vi "Begin_ConveyorV2.vi"() -> (0 "error out":errorcluster)   [LabVIEW 2012]
uses:
  <vilib>/Rock Robotics/SystemInterfaces/Typedef/FPGA_TypedefDigitalModule.ctl
  <vilib>/Rock Robotics/SystemInterfaces/DIO/FPGA_DIOChannel.ctl
  <vilib>/Rock Robotics/WPI/CAN/Jaguar/SubVIs/WPI_CANJaguar_BrakeCoastMode.ctl
  <vilib>/Rock Robotics/WPI/MotorControl/WPI_MotorControlOpenCANJaguar.vi
  <vilib>/Rock Robotics/SystemInterfaces/AI/FPGA_AIChannel.ctl
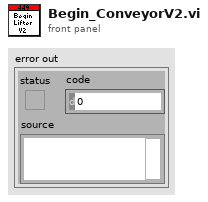
[diagram p1: front panel]
types:
  T1 = typedef "WPI_CANJaguar_BrakeCoastMode.ctl" = enum8{"Jumper", "Brake", "Coast"}
  T2 = typedef "WPI_MotorControlDeviceRef.ctl" = cluster{"DeviceStatus":errorcluster, "Type":enum16{"PWM", "CAN"}, "PWM":cluster{"Digital Module":T3, "PWM Channel":T4, "DeadBand":T5}, "CAN":cluster{"Device Number":u8, "Control Mode":T6, "Semaphore":T7, "Max Vout":dbl}, "Invert":bool, "TransformRef":T8, "InvTransformRef":T8}
  T3 = typedef "FPGA_TypedefDigitalModule.ctl" = enum16{"Digital Module 1", "Digital Module 2"}
  T4 = typedef "FPGA_DIOPWMChannel.ctl" = enum8{"PWM 1", "PWM 2", "PWM 3", "PWM 4", "PWM 5", "PWM 6", "PWM 7", "PWM 8", "PWM 9", "PWM 10", "Invalid"}
  T5 = typedef "WPI_PWMDeadband.ctl" = cluster{"Name":string, "maxPositivePwm":i32, "minPositivePwm":i32, "centerPwm":i32, "maxNegativePwm":i32, "minNegativePwm":i32, "angularRange":u16}
  T6 = typedef "WPI_CANJaguar_ControlMode.ctl" = enum8{"Percent VBus", "Current", "Speed", "Position", "Voltage"}
  T7 = typedef "Semaphore RefNum" = refnum<k1>
  T8 = typedef "WPI_PWMTransform_ConPane.ctl" = refnum<vi>
  T9 = typedef "FPGA_AIChannel.ctl" = enum8{"AI 1", "AI 2", "AI 3", "AI 4", "AI 5", "AI 6", "AI 7", "AI 8", "Invalid"}
  T10 = typedef "FPGA_DIOChannel.ctl" = enum8{"DIO 1", "DIO 2", "DIO 3", "DIO 4", "DIO 5", "DIO 6", "DIO 7", "DIO 8", "DIO 9", "DIO 10", "DIO 11", "DIO 12", "DIO 13", "DIO 14", "Invalid"}
  T11 = typedef "WPI_DigitalInputDevRef.ctl" = cluster{"DevStatus":errorcluster, "DIO Channel":T10, "Digital Module":T3}
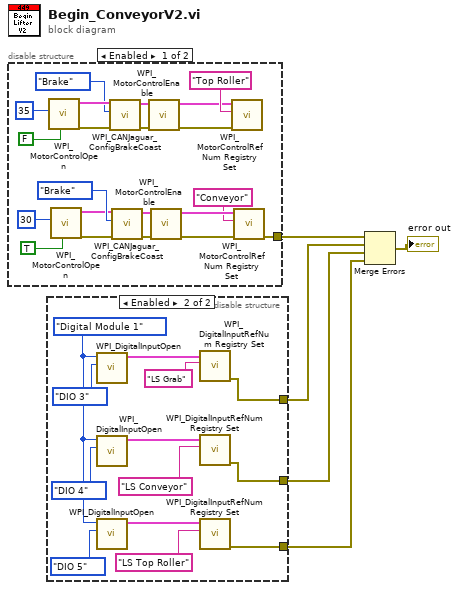
[diagram p0: block diagram]
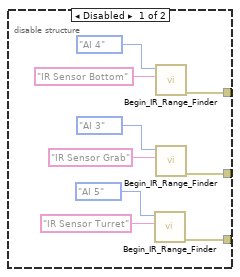
[diagram p2: hidden frame]
diagram:
  n1 = disable-structure shown="Enabled" {
    disable-tunnel: [w16 _] -> w4
    frame Enabled {
      n2 = call-poly <vilib>:"WPI_MotorControlOpen.vi"("Invert"=FALSE, "Device Number"=u8 35) -> ("error out"=w7:errorcluster, "MotorControlDeviceRef"=w8:T2)  [unwired: 8 in]
      n3 = call-poly <vilib>:"WPI_MotorControlOpen.vi"("Invert"=TRUE, "Device Number"=u8 30) -> ("error out"=w25:errorcluster, "MotorControlDeviceRef"=w24:T2)  [unwired: 8 in]
      n4 = call <vilib>:"WPI_CANJaguar_ConfigBrakeCoast.vi"("error in (no error)"=w7, "Brake / Coast Mode"=WPI_CANJaguar_BrakeCoastMode."Brake", "CAN Jaguar Ref"=w8) -> ("error out"=w10:errorcluster, "CAN Jaguar Ref Out"=w9:T2)  [unwired: 7 in]
      n5 = call <vilib>:"WPI_CANJaguar_ConfigBrakeCoast.vi"("error in (no error)"=w25, "Brake / Coast Mode"=WPI_CANJaguar_BrakeCoastMode."Brake", "CAN Jaguar Ref"=w24) -> ("error out"=w22:errorcluster, "CAN Jaguar Ref Out"=w23:T2)  [unwired: 7 in]
      n6 = call <vilib>:"WPI_MotorControlEnable.vi"("error in (no error)"=w10, "CAN Jaguar Ref"=w9) -> ("error out"=w15:errorcluster, "CAN Jaguar Ref Out"=w13:T2)  [unwired: 8 in]
      n7 = call <vilib>:"WPI_MotorControlEnable.vi"("error in (no error)"=w22, "CAN Jaguar Ref"=w23) -> ("error out"=w17:errorcluster, "CAN Jaguar Ref Out"=w19:T2)  [unwired: 8 in]
      n8 = call <vilib>:"WPI_MotorControlRefNum Registry Set.vi"("error in (no error)"=w15, "refnum name"="Top Roller", "MotorControlDevRef"=w13) -> ()  [unwired: 7 in, 2 out]
      n9 = call <vilib>:"WPI_MotorControlRefNum Registry Set.vi"("error in (no error)"=w17, "refnum name"="Conveyor", "MotorControlDevRef"=w19) -> ("error out"=w16:errorcluster)  [unwired: 7 in, 1 out]
    }
    frame Disabled {
    }
  }
  n10 = disable-structure shown="Enabled" {
    disable-tunnel: [w35 w44] -> w3
    disable-tunnel: [w34 w43] -> w2
    disable-tunnel: [w31 w42] -> w1
    frame Disabled {
      n11 = call "Begin_IR_Range_Finder.vi"("Reference Name"="IR Sensor Turret", "Analog Channel"=FPGA_AIChannel."AI 5") -> ("error out"=w31:errorcluster)  [unwired: 9 in]
      n12 = call "Begin_IR_Range_Finder.vi"("Reference Name"="IR Sensor Bottom", "Analog Channel"=FPGA_AIChannel."AI 4") -> ("error out"=w35:errorcluster)  [unwired: 9 in]
      n13 = call "Begin_IR_Range_Finder.vi"("Reference Name"="IR Sensor Grab", "Analog Channel"=FPGA_AIChannel."AI 3") -> ("error out"=w34:errorcluster)  [unwired: 9 in]
    }
    frame Enabled {
      w48 = FPGA_TypedefDigitalModule."Digital Module 1" ("Digital Module (Module 1)")
      n14 = call <vilib>:"WPI_DigitalInputOpen.vi"("DIO Channel"=FPGA_DIOChannel."DIO 3", "Digital Module (Module 1)"=w48) -> ("DigitalInputDevRef"=w46:T11)  [unwired: 8 in, 1 out]
      n15 = call <vilib>:"WPI_DigitalInputOpen.vi"("DIO Channel"=FPGA_DIOChannel."DIO 4", "Digital Module (Module 1)"=w48) -> ("DigitalInputDevRef"=w39:T11)  [unwired: 8 in, 1 out]
      n16 = call <vilib>:"WPI_DigitalInputOpen.vi"("DIO Channel"=FPGA_DIOChannel."DIO 5", "Digital Module (Module 1)"=w48) -> ("DigitalInputDevRef"=w38:T11)  [unwired: 8 in, 1 out]
      n17 = call <vilib>:"WPI_DigitalInputRefNum Registry Set.vi"("refnum name"="LS Grab", "DigitalInputDevRef"=w46) -> ("error out"=w44:errorcluster)  [unwired: 8 in, 1 out]
      n18 = call <vilib>:"WPI_DigitalInputRefNum Registry Set.vi"("refnum name"="LS Conveyor", "DigitalInputDevRef"=w39) -> ("error out"=w43:errorcluster)  [unwired: 8 in, 1 out]
      n19 = call <vilib>:"WPI_DigitalInputRefNum Registry Set.vi"("refnum name"="LS Top Roller", "DigitalInputDevRef"=w38) -> ("error out"=w42:errorcluster)  [unwired: 8 in, 1 out]
    }
  }
  n20 = Merge Errors(w4, w3, w2, w1) -> (→"error out":errorcluster)
